vi "4_VisualAD_HyperParam_Search.vi"() -> ()   [LabVIEW 2020]
uses:
  <vilib>/Ngene/DeepLTK Anomaly Detection Addon/Toolkit/API/Controls/NNPC_Coreset_Params.ctl
  <vilib>/Ngene/DeepLTK Anomaly Detection Addon/Toolkit/API/Controls/Distance_Metric.ctl
  <vilib>/Ngene/DeepLTK Anomaly Detection Addon/Toolkit/API/Controls/NNPC_Setup.ctl
  <vilib>/Ngene/Deep Learning Toolkit/Toolkit/NN_Data/API/NN_Dims(C,H,W).ctl
  <vilib>/Ngene/Deep Learning Toolkit/Toolkit/NN_Network/Controls/NN_Device.ctl
  <vilib>/Ngene/DeepLTK Anomaly Detection Addon/Toolkit/API/Controls/Feature_Scorer_Params.ctl
  <vilib>/Ngene/DeepLTK Anomaly Detection Addon/Toolkit/API/Controls/Gaussian_Blur.ctl
  <vilib>/Ngene/DeepLTK Anomaly Detection Addon/Toolkit/API/Controls/Evaluation_Metrics.ctl
  <vilib>/Ngene/DeepLTK Anomaly Detection Addon/Toolkit/API/Controls/Eval_Results.ctl
  <vilib>/Ngene/DeepLTK Anomaly Detection Addon/Toolkit/API/Controls/MinMax.ctl
  <vilib>/Ngene/DeepLTK Anomaly Detection Addon/Toolkit/API/Controls/NNPC_Random_Projection_CFG.ctl
  <vilib>/Ngene/DeepLTK Anomaly Detection Addon/Toolkit/API/Controls/Dim_Reduction_Method.ctl
  <vilib>/Ngene/DeepLTK Anomaly Detection Addon/Toolkit/API/Controls/NNFE_CFG.ctl
  <vilib>/Ngene/DeepLTK Anomaly Detection Addon/Toolkit/API/Controls/Layer_Selector.ctl
  <vilib>/Ngene/DeepLTK Anomaly Detection Addon/Toolkit/API/Controls/Feature_Layer_Selector.ctl
  <vilib>/Ngene/DeepLTK Anomaly Detection Addon/Toolkit/API/Controls/Interpolation_Selector.ctl
  subVIs/HyperParam_Search/Controls/Feature_Layers_CFG.ctl
  subVIs/HyperParam_Search/Controls/Model_Info_and_Report.ctl
  subVIs/Dataset_Reader/Controls/Read_Options.ctl
  <vilib>/Ngene/DeepLTK Anomaly Detection Addon/Toolkit/API/Controls/NNPC_PreProcessing_Options.ctl
  <vilib>/Ngene/DeepLTK Anomaly Detection Addon/Toolkit/API/Controls/Crop_CFG.ctl
  <vilib>/Ngene/DeepLTK Anomaly Detection Addon/Toolkit/API/Controls/NNPC_DS_Stats.ctl
  <vilib>/Ngene/DeepLTK Anomaly Detection Addon/Toolkit/API/Controls/Image_Stats_RGB.ctl
  <vilib>/Ngene/DeepLTK Anomaly Detection Addon/Toolkit/API/Controls/Eval_Config.ctl
  <vilib>/Ngene/DeepLTK Anomaly Detection Addon/Toolkit/API/NNPC_Generate_Embedding/NNPC_Generate_Embedding(Dataset).vi
  <vilib>/Ngene/DeepLTK Anomaly Detection Addon/Toolkit/API/NNPC_Predict/NNPC_Predict(Dataset).vi
  <vilib>/Ngene/Deep Learning Toolkit/Toolkit/NN_Data/subVIs/Dataset_Destroy/NN_Dataset_Destroy(In3D_Out3D).vi
  <vilib>/Ngene/DeepLTK Anomaly Detection Addon/Toolkit/DeepLTK_Anomaly_Detection_Addon.lvlib
  <vilib>/Ngene/Deep Learning Toolkit/Toolkit/Deep_Learning_Toolkit_by_Ngene.lvlib
panel:
  in  "Model_Info_and_Report":T1={"Idx"=0, "Name"="", "Feature Extractor"="wrn_50_2_2_bnmerge", "Layers"="", "DS_Size"=0, "H"=0, "W"=-1, "Coreset Size"=0, "Proj_Dim"=0, "Good_Max(Img)"=0.0, "Bad_Min(Img)"=0.0, "Rel_Margin"=0.0, "Image_AUC"=0.0, "Pixel_AUC"=0.0, "Image_F1_Max"=0.0, "Pixel_F1_Max"=0.0, "Train_Time"=0.0, "Inf_Time"=0.0} {"Rel_Margin" format="%#.5f"; "Bad_Min(Img)" format="%#.5f"; "Good_Max(Img)" format="%#.5f"; "Pixel_F1_Max" format="%#.5f"; "Pixel_AUC" format="%#.5f"; "Image_F1_Max" format="%#.5f"; "Image_AUC" format="%#.5f"}
  in  "Tab Control":enum32{"Setup", "Results"}(tab)
  in  "Min_Layers_In_Group":u16=1
  in  "Dataset_Path(Train/Test/GT)":path=path "D:/Ngene/GitHub/deepltk_examples/3_Image_Processing/36_Anomaly_Detection/Dataset/Playing_Cards_3ofHearts"
  in  "Destination_Path":path=path "D:/working"
  in  "Coreset_Size":sgl[](array[numeric])=[5000.0, 10000.0, 15000.0]
  in  "Proj._Dim.":i32[](array[numeric])=[-1]
  in  "Coreset_Params":T2={"Distance_Metric"=enum."Euclidean", "CoreSet_Size"=1.0, "Start_idx"=3}
  in  "NNPC_Setup":T4={"Input_Dims"={"C"=3, "H"=224, "W"=224}, "mBatch"=1, "Device"=enum."GPU", "GPU Id"=0}
  in  "Feature_Scorer_Params":T7={"Nearest_Neighbors"=1, "Calculate Anomaly Map"=FALSE, "Gaussian_Blur"={"Kernel_Size"=33, "Sigma"=4.0}}
  in  "Dim Reduction":T9={"Method"=enum."Rnd_Proj", "Target_Dim"=-1, "Seed"=42}
  in  "NNFE_CFG":T11={"Name"="Cards_3ofHearts", "Layer_Selection_By"=enum."Stride", "Feature_Layers"={"[LayerID, PatchSize]"=[{"Layer_ID"=8, "Patch_Size"=3}, {"Layer_ID"=16, "Patch_Size"=3}]}, "Interpolation_Type"=enum."Bi-Linear"}
  in  "NNFE_Folder_Paths":path[](array[path])=[path "D:/Ngene/GitHub/deepltk_examples/3_Image_Processing/36_Anomaly_Detection/NNFE/WRN_50_2_2_L3"]
  in  "Patch Sizes":i32[](array[numeric])=[1, 3, 5]
  in  "Layer ID":i32[](array[numeric])=[4, 8, 16]
  out "Generated_Feature_Layers":T13[](array[typedef])=[{"[LayerID, PatchSize]"=[{"Layer_ID"=16, "Patch_Size"=1}]}, {"[LayerID, PatchSize]"=[{"Layer_ID"=16, "Patch_Size"=3}]}, {"[LayerID, PatchSize]"=[{"Layer_ID"=16, "Patch_Size"=5}]}, {"[LayerID, PatchSize]"=[{"Layer_ID"=8, "Patch_Size"=1}]}, {"[LayerID, PatchSize]"=[{"Layer_ID"=8, "Patch_Size"=1}, {"Layer_ID"=16, "Patch_Size"=1}]}, {"[LayerID, PatchSize]"=[{"Layer_ID"=8, "Patch_Size"=1}, {"Layer_ID"=16, "Patch_Size"=3}]}, {"[LayerID, PatchSize]"=[{"Layer_ID"=8, "Patch_Size"=1}, {"Layer_ID"=16, "Patch_Size"=5}]}, {"[LayerID, PatchSize]"=[{"Layer_ID"=8, "Patch_Size"=3}]}, {"[LayerID, PatchSize]"=[{"Layer_ID"=8, "Patch_Size"=3}, {"Layer_ID"=16, "Patch_Size"=1}]}, {"[LayerID, PatchSize]"=[{"Layer_ID"=8, "Patch_Size"=3}, {"Layer_ID"=16, "Patch_Size"=3}]}, {"[LayerID, PatchSize]"=[{"Layer_ID"=8, "Patch_Size"=3}, {"Layer_ID"=16, "Patch_Size"=5}]}, {"[LayerID, PatchSize]"=[{"Layer_ID"=8, "Patch_Size"=5}]}, {"[LayerID, PatchSize]"=[{"Layer_ID"=8, "Patch_Size"=5}, {"Layer_ID"=16, "Patch_Size"=1}]}, {"[LayerID, PatchSize]"=[{"Layer_ID"=8, "Patch_Size"=5}, {"Layer_ID"=16, "Patch_Size"=3}]}, {"[LayerID, PatchSize]"=[{"Layer_ID"=8, "Patch_Size"=5}, {"Layer_ID"=16, "Patch_Size"=5}]}, {"[LayerID, PatchSize]"=[{"Layer_ID"=4, "Patch_Size"=1}]}, {"[LayerID, PatchSize]"=[{"Layer_ID"=4, "Patch_Size"=1}, {"Layer_ID"=16, "Patch_Size"=1}]}, {"[LayerID, PatchSize]"=[{"Layer_ID"=4, "Patch_Size"=1}, {"Layer_ID"=16, "Patch_Size"=3}]}, {"[LayerID, PatchSize]"=[{"Layer_ID"=4, "Patch_Size"=1}, {"Layer_ID"=16, "Patch_Size"=5}]}, {"[LayerID, PatchSize]"=[{"Layer_ID"=4, "Patch_Size"=1}, {"Layer_ID"=8, "Patch_Size"=1}]}, {"[LayerID, PatchSize]"=[{"Layer_ID"=4, "Patch_Size"=1}, {"Layer_ID"=8, "Patch_Size"=3}]}, {"[LayerID, PatchSize]"=[{"Layer_ID"=4, "Patch_Size"=1}, {"Layer_ID"=8, "Patch_Size"=5}]}, {"[LayerID, PatchSize]"=[{"Layer_ID"=4, "Patch_Size"=3}]}, {"[LayerID, PatchSize]"=[{"Layer_ID"=4, "Patch_Size"=3}, {"Layer_ID"=16, "Patch_Size"=1}]}, {"[LayerID, PatchSize]"=[{"Layer_ID"=4, "Patch_Size"=3}, {"Layer_ID"=16, "Patch_Size"=3}]}, {"[LayerID, PatchSize]"=[{"Layer_ID"=4, "Patch_Size"=3}, {"Layer_ID"=16, "Patch_Size"=5}]}, {"[LayerID, PatchSize]"=[{"Layer_ID"=4, "Patch_Size"=3}, {"Layer_ID"=8, "Patch_Size"=1}]}, {"[LayerID, PatchSize]"=[{"Layer_ID"=4, "Patch_Size"=3}, {"Layer_ID"=8, "Patch_Size"=3}]}, {"[LayerID, PatchSize]"=[{"Layer_ID"=4, "Patch_Size"=3}, {"Layer_ID"=8, "Patch_Size"=5}]}, {"[LayerID, PatchSize]"=[{"Layer_ID"=4, "Patch_Size"=5}]}, {"[LayerID, PatchSize]"=[{"Layer_ID"=4, "Patch_Size"=5}, {"Layer_ID"=16, "Patch_Size"=1}]}, {"[LayerID, PatchSize]"=[{"Layer_ID"=4, "Patch_Size"=5}, {"Layer_ID"=16, "Patch_Size"=3}]}, {"[LayerID, PatchSize]"=[{"Layer_ID"=4, "Patch_Size"=5}, {"Layer_ID"=16, "Patch_Size"=5}]}, {"[LayerID, PatchSize]"=[{"Layer_ID"=4, "Patch_Size"=5}, {"Layer_ID"=8, "Patch_Size"=1}]}, {"[LayerID, PatchSize]"=[{"Layer_ID"=4, "Patch_Size"=5}, {"Layer_ID"=8, "Patch_Size"=3}]}, {"[LayerID, PatchSize]"=[{"Layer_ID"=4, "Patch_Size"=5}, {"Layer_ID"=8, "Patch_Size"=5}]}]
  in  "Max_Layers_In_Group":u16=2
  out "error out":errorcluster
  in  "Img Res. H":i32[](array[numeric])=[224, 368]
  in  "Img Res. W":i32[](array[numeric])=[224, 368]
  in  "Single DS?":bool=TRUE
  out "Img._W":i32=224
  out "Elapsed Time":dbl=22.38694479999998 format="%<%H:%M:%S>t"
  out "Max_Dist":sgl[](graph)
  out "Tot Itr of one DS":i32=216
  out "Current Iter":i32=12
  out "Coreset Size":i32=3
  out "Proj. Dim.":i32=1
  out "Img Res.":i32=2
  out "Feature_Layers":i32=36
  out "Elapsed Time":dbl=22.38694479999998
  out "Evaluation_Metrics(Image)":T15={"Scores(Good)"={"X Values"=[56.569074115753175, 56.90936315536499, 57.249652194976804, 57.58994123458862, 57.93023027420044, 58.27051931381226, 58.610808353424076, 58.95109739303589, 59.291386432647705, 59.63167547225952, 59.971964511871334, 60.31225355148315, 60.65254259109497, 60.99283163070679, 61.33312067031861, 61.67340970993042, 62.013698749542236, 62.353987789154054, 62.694276828765865, 63.03456586837768, 63.3748549079895, 63.71514394760132, 64.05543298721314, 64.39572202682496, 64.73601106643676, 65.07630010604859, 65.4165891456604, 65.75687818527223, 66.09716722488403, 66.43745626449585, 66.77774530410767, 67.11803434371947, 67.4583233833313, 67.79861242294311, 68.13890146255494, 68.47919050216674, 68.81947954177856, 69.15976858139038, 69.50005762100218, 69.84034666061402, 70.18063570022582, 70.52092473983765, 70.86121377944946, 71.20150281906129, 71.5417918586731, 71.88208089828491, 72.22236993789673, 72.56265897750853, 72.90294801712037, 73.24323705673217, 73.583526096344, 73.9238151359558, 74.26410417556762, 74.60439321517944, 74.94468225479126, 75.28497129440308, 75.62526033401488, 75.96554937362671, 76.30583841323852, 76.64612745285035, 76.98641649246215, 77.32670553207397, 77.66699457168579, 78.0072836112976, 78.34757265090943, 78.68786169052123, 79.02815073013306, 79.36843976974487, 79.7087288093567, 80.0490178489685, 80.38930688858032, 80.72959592819214, 81.06988496780394, 81.41017400741578, 81.75046304702758, 82.09075208663941, 82.43104112625122, 82.77133016586303, 83.11161920547485, 83.45190824508667, 83.79219728469849, 84.13248632431029, 84.47277536392212, 84.81306440353393, 85.15335344314576, 85.49364248275756, 85.83393152236938, 86.1742205619812, 86.514509601593, 86.85479864120484, 87.19508768081664, 87.53537672042847, 87.87566576004028, 88.2159547996521, 88.55624383926391, 88.89653287887573, 89.23682191848755, 89.57711095809937, 89.91739999771119, 90.25768903732299], "Histogram: h(x)"=[3, 0, 0, 0, 1, 0, 1, 1, 1, 2, 1, 0, 0, 1, 0, 0, 3, 2, 0, 0, 0, 1, 0, 1, 0, 0, 0, 0, 0, 0, 0, 0, 0, 0, 0, 0, 0, 0, 0, 0, 0, 0, 0, 1, 1, 0, 0, 0, 0, 0, 0, 0, 0, 0, 0, 0, 0, 0, 0, 1, 0, 0, 0, 0, 0, 0, 0, 0, 0, 1, 0, 0, 0, 0, 0, 0, 0, 0, 0, 0, 0, 1, 1, 0, 0, 1, 0, 0, 0, 0, 0, 0, 0, 0, 0, 0, 0, 0, 0, 0]}, "Scores(Bad)"={"X Values"=[56.569074115753175, 56.90936315536499, 57.249652194976804, 57.58994123458862, 57.93023027420044, 58.27051931381226, 58.610808353424076, 58.95109739303589, 59.291386432647705, 59.63167547225952, 59.971964511871334, 60.31225355148315, 60.65254259109497, 60.99283163070679, 61.33312067031861, 61.67340970993042, 62.013698749542236, 62.353987789154054, 62.694276828765865, 63.03456586837768, 63.3748549079895, 63.71514394760132, 64.05543298721314, 64.39572202682496, 64.73601106643676, 65.07630010604859, 65.4165891456604, 65.75687818527223, 66.09716722488403, 66.43745626449585, 66.77774530410767, 67.11803434371947, 67.4583233833313, 67.79861242294311, 68.13890146255494, 68.47919050216674, 68.81947954177856, 69.15976858139038, 69.50005762100218, 69.84034666061402, 70.18063570022582, 70.52092473983765, 70.86121377944946, 71.20150281906129, 71.5417918586731, 71.88208089828491, 72.22236993789673, 72.56265897750853, 72.90294801712037, 73.24323705673217, 73.583526096344, 73.9238151359558, 74.26410417556762, 74.60439321517944, 74.94468225479126, 75.28497129440308, 75.62526033401488, 75.96554937362671, 76.30583841323852, 76.64612745285035, 76.98641649246215, 77.32670553207397, 77.66699457168579, 78.0072836112976, 78.34757265090943, 78.68786169052123, 79.02815073013306, 79.36843976974487, 79.7087288093567, 80.0490178489685, 80.38930688858032, 80.72959592819214, 81.06988496780394, 81.41017400741578, 81.75046304702758, 82.09075208663941, 82.43104112625122, 82.77133016586303, 83.11161920547485, 83.45190824508667, 83.79219728469849, 84.13248632431029, 84.47277536392212, 84.81306440353393, 85.15335344314576, 85.49364248275756, 85.83393152236938, 86.1742205619812, 86.514509601593, 86.85479864120484, 87.19508768081664, 87.53537672042847, 87.87566576004028, 88.2159547996521, 88.55624383926391, 88.89653287887573, 89.23682191848755, 89.57711095809937, 89.91739999771119, 90.25768903732299], "Histogram: h(x)"=[0, 0, 0, 0, 0, 0, 0, 0, 0, 0, 0, 0, 0, 0, 0, 0, 0, 0, 0, 0, 0, 0, 0, 0, 0, 0, 0, 0, 0, 0, 0, 0, 0, 0, 0, 0, 0, 0, 0, 0, 0, 0, 0, 0, 0, 0, 0, 0, 0, 0, 0, 0, 0, 0, 0, 0, 0, 0, 0, 0, 0, 0, 1, 0, 0, 0, 1, 0, 0, 2, 0, 0, 3, 1, 2, 0, 2, 0, 1, 1, 1, 0, 2, 3, 2, 1, 0, 0, 0, 1, 0, 0, 0, 0, 0, 0, 0, 0, 0, 1]}, "Eval Stats"={"Scores(Good)"={"Min"=56.39893, "Max"=85.355675}, "Scores(Bad)"={"Min"=77.81394, "Max"=90.42783}, "# of Samples(Good)"=25, "# of Samples(Bad)"=25, "AUROC"=0.9096, "F1_Max"=0.92592597, "Thrshld(F1_Max)"=76.63233, "Prec.(F1_Max)"=0.86206895, "Recall(F1_Max)"=1.0, "FPR(F1_Max)"=0.16, "FNR(F1_Max)"=0.0}} {"Eval Stats"."Recall(F1_Max)" format="%#.5f"; "Eval Stats"."FPR(F1_Max)" format="%#.5f"; "Eval Stats"."FNR(F1_Max)" format="%#.5f"; "Eval Stats"."Prec.(F1_Max)" format="%#.5f"; "Eval Stats"."F1_Max" format="%#.5f"; "Eval Stats"."AUROC" format="%#.5f"; "Eval Stats"."Scores(Bad)"."Min" format="%#_5g"; "Eval Stats"."Scores(Good)"."Min" format="%#_5g"; "Eval Stats"."Thrshld(F1_Max)" format="%#_5f"}
  out "Evaluation_Metrics(Pixel)":T15={"Scores(Good)"={"X Values"=[0.0, 0.0, 0.0, 0.0, 0.0, 0.0, 0.0, 0.0, 0.0, 0.0, 0.0, 0.0, 0.0, 0.0, 0.0, 0.0, 0.0, 0.0, 0.0, 0.0, 0.0, 0.0, 0.0, 0.0, 0.0, 0.0, 0.0, 0.0, 0.0, 0.0, 0.0, 0.0, 0.0, 0.0, 0.0, 0.0, 0.0, 0.0, 0.0, 0.0, 0.0, 0.0, 0.0, 0.0, 0.0, 0.0, 0.0, 0.0, 0.0, 0.0, 0.0, 0.0, 0.0, 0.0, 0.0, 0.0, 0.0, 0.0, 0.0, 0.0, 0.0, 0.0, 0.0, 0.0, 0.0, 0.0, 0.0, 0.0, 0.0, 0.0, 0.0, 0.0, 0.0, 0.0, 0.0, 0.0, 0.0, 0.0, 0.0, 0.0, 0.0, 0.0, 0.0, 0.0, 0.0, 0.0, 0.0, 0.0, 0.0, 0.0, 0.0, 0.0, 0.0, 0.0, 0.0, 0.0, 0.0, 0.0, 0.0, 0.0], "Histogram: h(x)"=[]}, "Scores(Bad)"={"X Values"=[], "Histogram: h(x)"=[]}, "Eval Stats"={"Scores(Good)"={"Min"=0.0, "Max"=0.0}, "Scores(Bad)"={"Min"=0.0, "Max"=0.0}, "# of Samples(Good)"=0, "# of Samples(Bad)"=0, "AUROC"=-1.0, "F1_Max"=0.0, "Thrshld(F1_Max)"=0.0, "Prec.(F1_Max)"=0.0, "Recall(F1_Max)"=0.0, "FPR(F1_Max)"=0.0, "FNR(F1_Max)"=0.0}} {"Eval Stats"."Recall(F1_Max)" format="%#.5f"; "Eval Stats"."FPR(F1_Max)" format="%#.5f"; "Eval Stats"."FNR(F1_Max)" format="%#.5f"; "Eval Stats"."Prec.(F1_Max)" format="%#.5f"; "Eval Stats"."F1_Max" format="%#.5f"; "Eval Stats"."AUROC" format="%#.5f"; "Eval Stats"."Scores(Bad)"."Min" format="%#_5g"; "Eval Stats"."Scores(Good)"."Min" format="%#_5g"; "Eval Stats"."Thrshld(F1_Max)" format="%#_5f"}
  out "Coreset Size":i32
  out "Coreset Size":i32=15000
  out "Proj. Dim.":i32=-1
  out "Img._H":i32=224
  out "Proj. Dim.":i32
  out "Img Res.":i32
  out "dT_Eval":dbl=0.00020089999998162966 format="%#_4p"
  out "dT_Inference":dbl=0.007889208000001417 format="%#_4p"
  out "dT_Coreset":dbl=11.027360000000044 format="%#_4p"
  out "dT_Embed":dbl=0.20192650000001322 format="%#_3p"
  out "dT_Init":dbl=0.13968869999996514 format="%#_3p"
  out "dT_DS_Read(Test)":dbl=0.14549890000000687 format="%#_3p"
  out "dT_DS_Read(Train)":dbl=0.19376790000001165 format="%#_3p"
  out "DS Size(Test)":i32=50
  out "DS Size(Train)":i32=50
  out "Feature_Layers":i32=4
  out "dT_DS_Read(Train)":dbl=0.19376790000001165 format="%#.0f"
  out "dT_DS_Read(Test)":dbl=0.14549890000000687 format="%#.0f"
  out "dT_Init":dbl=1.64397120000001 format="%#.0f"
  out "dT_Predict":dbl=2.67796850000002 format="%#.0f"
  out "dT_Coreset":dbl=16.00583629999994 format="%#.0f"
  out "dT_Embed":dbl=0.9169715000000451 format="%#.0f"
  out "dT_Eval":dbl=0.0023649000001455533 format="%#.0f"
  out "Feature Extractor":string="wrn_50_2_2_bnmerge"
  out "dT_Predict":dbl=0.3944604000000709 format="%#_5p"
  out "[LayerID, PatchSize]":T18=[{"Layer_ID"=8, "Patch_Size"=1}, {"Layer_ID"=16, "Patch_Size"=1}]
  in  "Stop":bool
  out "NNFE":i32
  out "NNFE":i32=1
  out "Best_Model":string="9_wrn_50_2_2_bnmerge_Res224x224_L8P1_Prj-1_CSet15k"
  out "Best_AUC":sgl=0.9696 format="%#_5g"
  out "DS":i32=1
  out "DS":i32
  out "DS_Name":string="Playing_Cards_3ofHearts"
  out "Crrnt Iter":i32=12
  out "Total Iters":i32=216
  out "Online_CoreSet_Size":sgl=-1.0 format="%#_4g"
  # "Total Iterations"
  # "Current Iteration"
  # "Current Settings"
  # "Total Times"
  # "Best Settings"
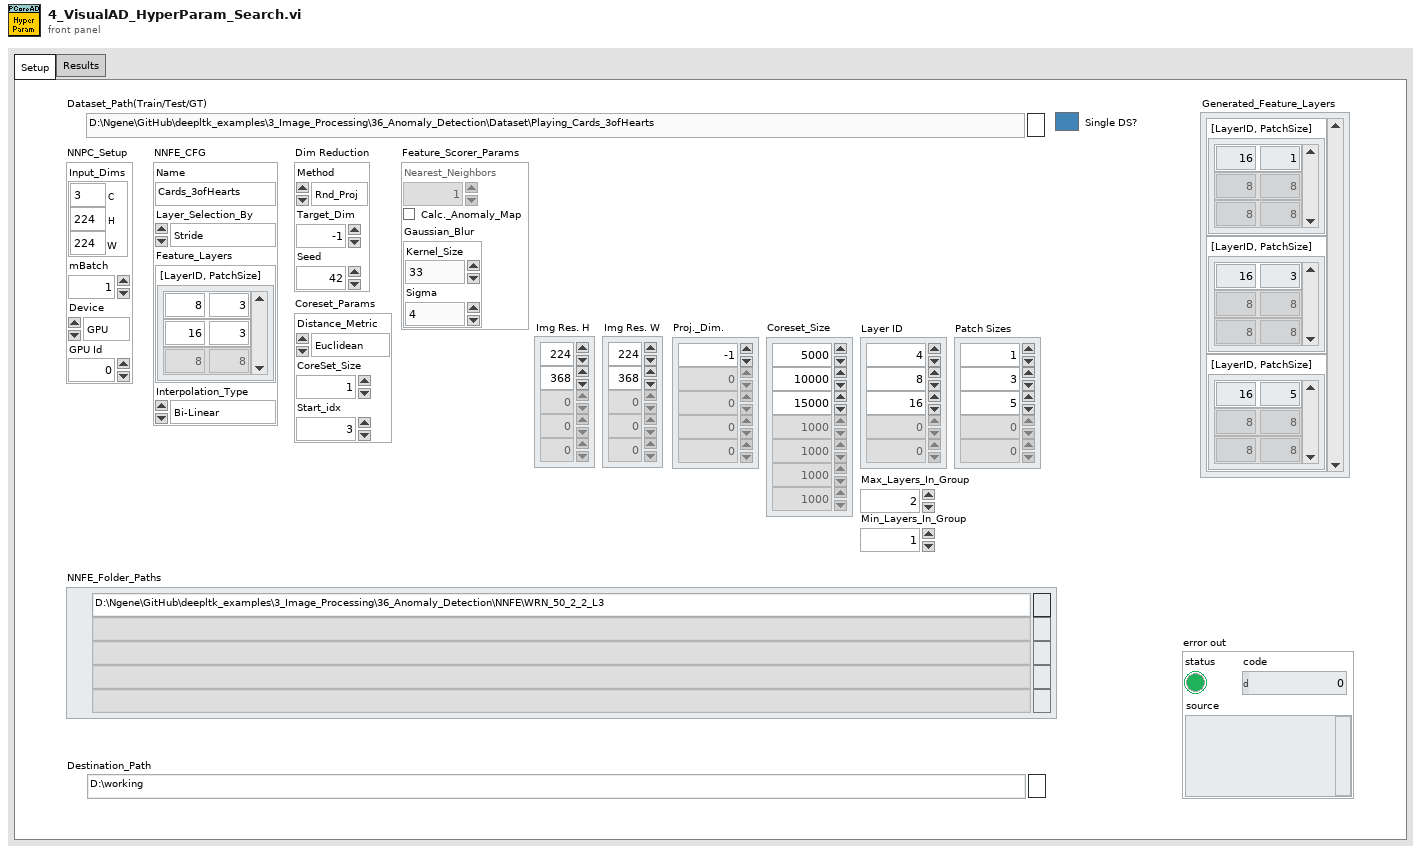
[diagram p1: front panel]
types:
  T1 = typedef "Model_Info_and_Report.ctl" = cluster{"Idx":i32, "Name":string, "Feature Extractor":string, "Layers":string, "DS_Size":i32, "H":i32, "W":i32, "Coreset Size":i32, "Proj_Dim":i32, "Good_Max(Img)":sgl, "Bad_Min(Img)":sgl, "Rel_Margin":sgl, "Image_AUC":sgl, "Pixel_AUC":sgl, "Image_F1_Max":sgl, "Pixel_F1_Max":sgl, "Train_Time":dbl, "Inf_Time":dbl}
  T2 = typedef "DeepLTK_Anomaly_Detection_Addon.lvlib/NNPC_Coreset_Params.ctl" = cluster{"Distance_Metric":T3, "CoreSet_Size":sgl, "Start_idx":i32}
  T3 = typedef "DeepLTK_Anomaly_Detection_Addon.lvlib/Distance_Metric.ctl" = enum16{"Euclidean", "Cosine"}
  T4 = typedef "DeepLTK_Anomaly_Detection_Addon.lvlib/NNPC_Setup.ctl" = cluster{"Input_Dims":T5, "mBatch":i32, "Device":T6, "GPU Id":i32}
  T5 = typedef "Deep_Learning_Toolkit_by_Ngene.lvlib/NN_Dims(C,H,W).ctl" = cluster{"C":i32, "H":i32, "W":i32}
  T6 = typedef "Deep_Learning_Toolkit_by_Ngene.lvlib/NN_Device.ctl" = enum16{"CPU", "GPU"}
  T7 = typedef "DeepLTK_Anomaly_Detection_Addon.lvlib/Feature_Scorer_Params.ctl" = cluster{"Nearest_Neighbors":i32, "Calculate Anomaly Map":bool, "Gaussian_Blur":T8}
  T8 = typedef "DeepLTK_Anomaly_Detection_Addon.lvlib/Gaussian_Blur.ctl" = cluster{"Kernel_Size":i32, "Sigma":sgl}
  T9 = typedef "DeepLTK_Anomaly_Detection_Addon.lvlib/NNPC_Random_Projection_CFG.ctl" = cluster{"Method":T10, "Target_Dim":i32, "Seed":i32}
  T10 = typedef "DeepLTK_Anomaly_Detection_Addon.lvlib/Dim_Reduction_Method.ctl" = enum16{"None", "Rnd_Proj", "PCA"}
  T11 = typedef "DeepLTK_Anomaly_Detection_Addon.lvlib/NNFE_CFG.ctl" = cluster{"Name":string, "Layer_Selection_By":T12, "Feature_Layers":T13, "Interpolation_Type":T14}
  T12 = typedef "DeepLTK_Anomaly_Detection_Addon.lvlib/Layer_Selector.ctl" = enum16{"Stride", "Layer_Idx"}
  T13 = typedef "DeepLTK_Anomaly_Detection_Addon.lvlib/Feature_Layer_Selector.ctl" = cluster{"[LayerID, PatchSize]":cluster{"Layer_ID":i32, "Patch_Size":i32}[]}
  T14 = typedef "DeepLTK_Anomaly_Detection_Addon.lvlib/Interpolation_Selector.ctl" = enum16{"Nearest", "Bi-Linear"}
  T15 = typedef "DeepLTK_Anomaly_Detection_Addon.lvlib/Evaluation_Metrics.ctl" = cluster{"Scores(Good)":cluster{"X Values":dbl[], "Histogram: h(x)":i32[]}, "Scores(Bad)":cluster{"X Values":dbl[], "Histogram: h(x)":i32[]}, "Eval Stats":T16}
  T16 = typedef "DeepLTK_Anomaly_Detection_Addon.lvlib/Eval_Results.ctl" = cluster{"Scores(Good)":T17, "Scores(Bad)":T17, "# of Samples(Good)":i32, "# of Samples(Bad)":i32, "AUROC":sgl, "F1_Max":sgl, "Thrshld(F1_Max)":sgl, "Prec.(F1_Max)":sgl, "Recall(F1_Max)":sgl, "FPR(F1_Max)":sgl, "FNR(F1_Max)":sgl}
  T17 = typedef "DeepLTK_Anomaly_Detection_Addon.lvlib/MinMax.ctl" = cluster{"Min":sgl, "Max":sgl}
  T18 = typedef "Feature_Layers_CFG.ctl" = cluster{"Layer_ID":i32, "Patch_Size":i32}[]
  T19 = typedef "DeepLTK_Anomaly_Detection_Addon.lvlib/NN_Paths.ctl" = cluster{"CFG":path, "BIN":path}
  T20 = enum16{"open", "replace", "create", "open or create", "replace or create", "replace or create with confirmation"}
  T21 = typedef "DeepLTK_Anomaly_Detection_Addon.lvlib/NNPC_PreProcessing_Options.ctl" = cluster{"DS_Name":string, "Input_Dims":T5, "Cropping":T22, "Interpolation Type":u32, "MultiStage_ReSample?":bool, "Dataset_Stats":T23}
  T22 = typedef "DeepLTK_Anomaly_Detection_Addon.lvlib/Crop_CFG.ctl" = cluster{"Left":sgl, "Top":sgl, "Right":sgl, "Bottom":sgl}
  T23 = typedef "DeepLTK_Anomaly_Detection_Addon.lvlib/NNPC_DS_Stats.ctl" = cluster{"means":T24, "stds":T24}
  T24 = typedef "DeepLTK_Anomaly_Detection_Addon.lvlib/Image_Stats_RGB.ctl" = cluster{"R":sgl, "G":sgl, "B":sgl}
  T25 = typedef "Read_Options.ctl" = cluster{"Read Bads?":bool, "Read GTs?":bool, "Update. DS Stats?":bool}
  T26 = typedef "DeepLTK_Anomaly_Detection_Addon.lvlib/Eval_Config.ctl" = cluster{"Extract_Good_Pixels_from_Bad":bool, "# bins":i32}
  T27 = typedef "Deep_Learning_Toolkit_by_Ngene.lvlib/NN_DataSet(In3D_Out3D).ctl" = cluster{"Dataset_Size":i32, "Dims_In":T5, "Labels":string[], "File Paths":path[], "Outputs Ref.":T28, "Inputs Ref.":variant, "Dims_Out":T5, "Custom_Data":variant}
  T28 = typedef "Deep_Learning_Toolkit_by_Ngene.lvlib/NN_Data_ref(4D_SGL).ctl" = refnum<data-value>
  T29 = typedef "DeepLTK_Anomaly_Detection_Addon.lvlib/NNPC_Instance.ctl" = cluster{"Name":string, "NN":T30, "MemBank_Data":T44}
  T30 = typedef "Deep_Learning_Toolkit_by_Ngene.lvlib/NN.ctl" = cluster{"Name":string, "No of Layers":i32, "mBatch":i32, "Layers":T31[], "Dimty":T32, "Dims_In":T5, "Dims_Out":T5, "Working_Dir":path, "Train?":bool, "Train_Params":T33, "LR_Update_Policy":T36, "Session Data":T38, "Ground_truth":T39, "NNg_hdls":T40, "NN_Device":T6, "GPU Id":i32, "Labels":string[], "Loss_Type":T41, "Loss_Cfg_Prms":variant, "NNG_WS":T42, "DryRun?":bool}
  T31 = typedef "Deep_Learning_Toolkit_by_Ngene.lvlib/NN_Layer_ref.ctl" = refnum<file>
  T32 = typedef "Deep_Learning_Toolkit_by_Ngene.lvlib/NN_In_Out_Dim-ty.ctl" = enum8{"In1D_Out1D", "In3D_Out1D", "In3D_Out3D", "In3D_OutBBox"}
  T33 = typedef "Deep_Learning_Toolkit_by_Ngene.lvlib/NN_Train_Params.ctl" = cluster{"Optimizer":T34, "Beta_1":sgl, "Beta_2":sgl, "Weight Decay(L1)":sgl, "Weight Decay(L2)":sgl, "Data_Sampling":T35}
  T34 = typedef "Deep_Learning_Toolkit_by_Ngene.lvlib/NN_Train_Optimizer.ctl" = enum16{"SGD", "Adam", "Adagrad", "Adadelta", "RMSProp", "Nesterov"}
  T35 = typedef "Deep_Learning_Toolkit_by_Ngene.lvlib/NN_Train_Data_Sampling.ctl" = enum16{"Random", "Sequential"}
  T36 = typedef "Deep_Learning_Toolkit_by_Ngene.lvlib/NN_LR_Policy_Cfg.ctl" = cluster{"Policy_Type":T37, "LR0":dbl, "k":sgl, "WarmUp_Policy":enum16{"Step", "Ramp"}, "WarmUp_Iter":i32, "WarmUp_Ratio":sgl}
  T37 = typedef "Deep_Learning_Toolkit_by_Ngene.lvlib/NN_LR_Policy_Type.ctl" = enum16{"Manual", "Step", "Exp", "1/t"}
  T38 = typedef "Deep_Learning_Toolkit_by_Ngene.lvlib/NN_Train_Session_Data.ctl" = cluster{"Epochs":sgl, "Tot_Iter":i32, "LR":sgl, "LR_iter":i32}
  T39 = typedef "Deep_Learning_Toolkit_by_Ngene.lvlib/NN_Ground_truth.ctl" = cluster{"Y":variant}
  T40 = typedef "Deep_Learning_Toolkit_by_Ngene.lvlib/nng_cuda_handles.ctl" = cluster{"cudnn":u64, "cublas":u64, "stream":u64, "curand":u64}
  T41 = typedef "Deep_Learning_Toolkit_by_Ngene.lvlib/NN_Loss_Type.ctl" = enum16{"None", "MSE", "CrossEntropy", "YOLO_v2", "YOLO_v4"}
  T42 = typedef "Deep_Learning_Toolkit_by_Ngene.lvlib/NNG_WS.ctl" = cluster{"NNG_WS_Mem":T43, "Max_WS_Size":i64}
  T43 = typedef "Deep_Learning_Toolkit_by_Ngene.lvlib/NNg_WS_Mem_DVR.ctl" = refnum<data-value>
  T44 = typedef "DeepLTK_Anomaly_Detection_Addon.lvlib/MemBank_and_Norm_Variants.ctl" = cluster{"MemBank":variant, "MemBank Norm":variant}
  T45 = typedef "DeepLTK_Anomaly_Detection_Addon.lvlib/Evaluation_Metrics(Pixel_Image).ctl" = cluster{"Evaluation_Metrics(Pixel)":T15, "Evaluation_Metrics(Image)":T15}
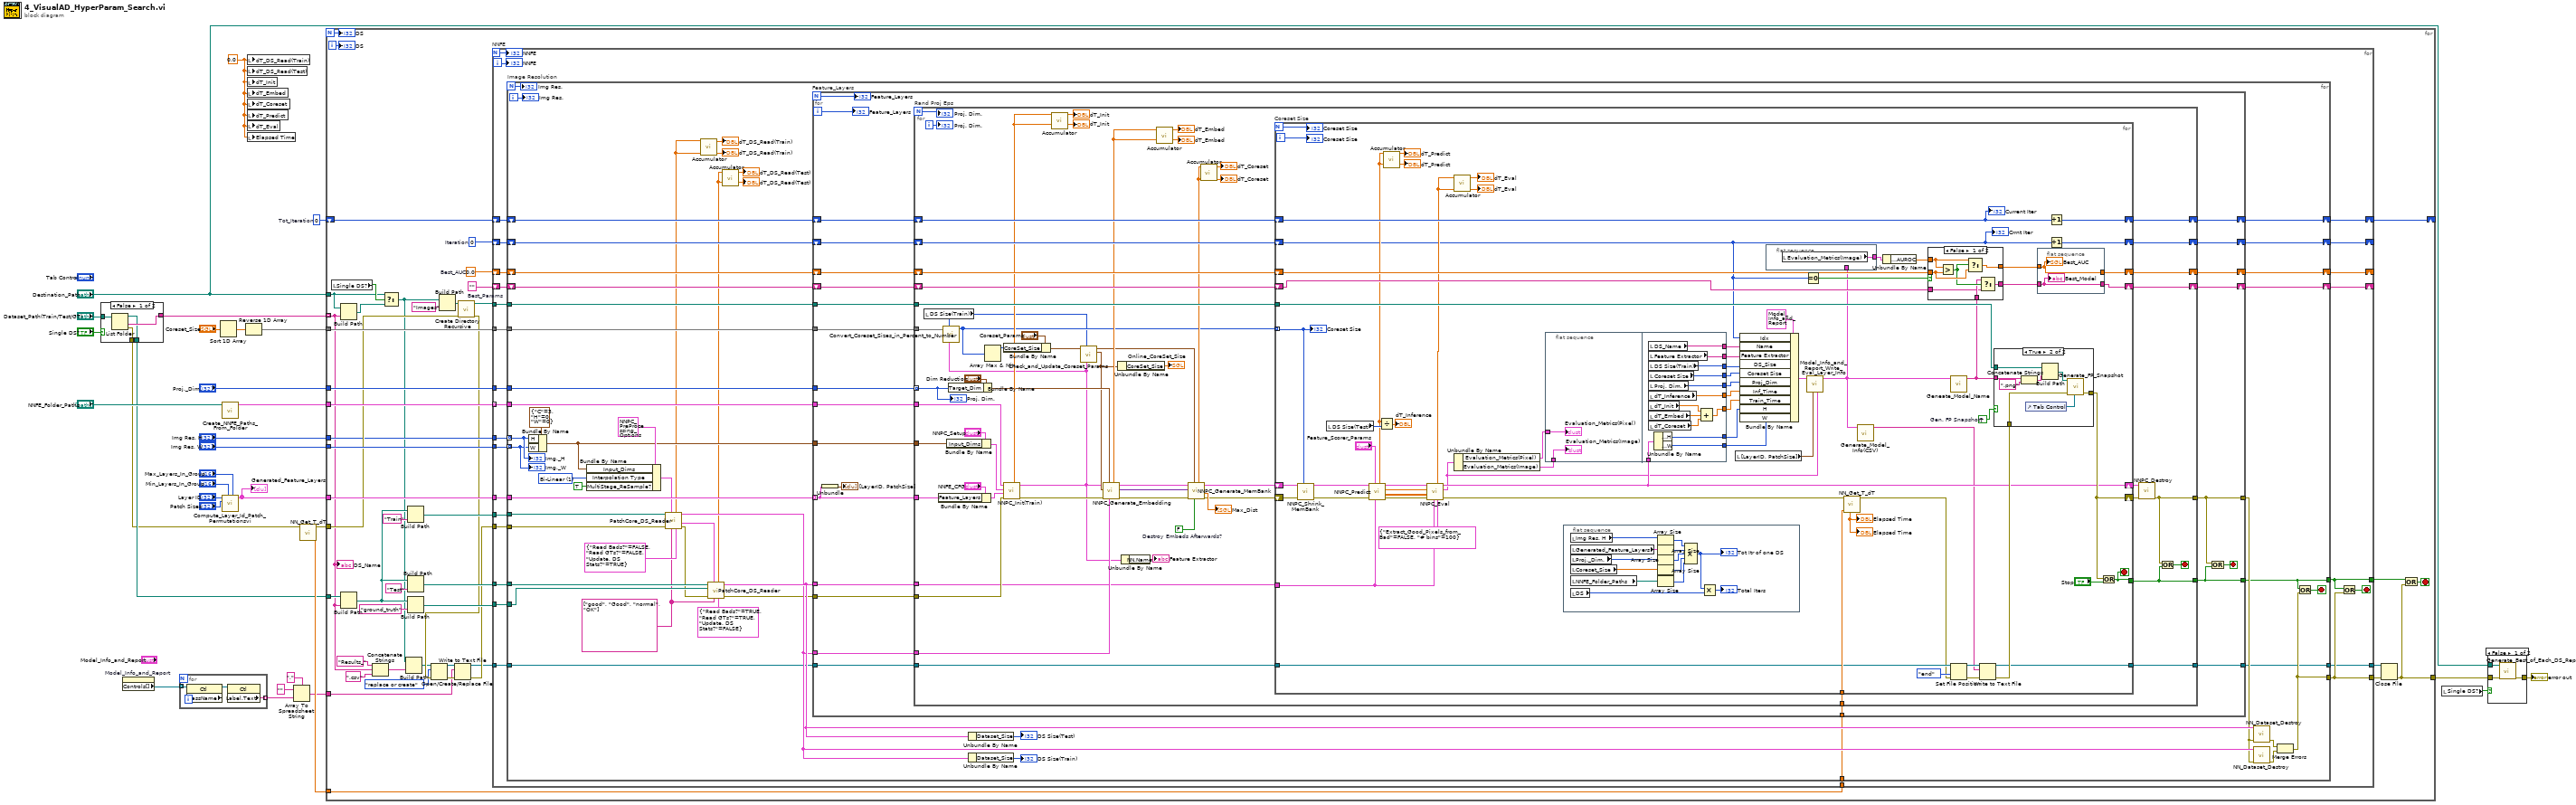
[diagram p0: block diagram]
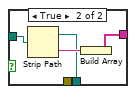
[diagram p4: hidden frame]
diagram:
  w10 = 0.0 ("dT_Eval")
  w20 = 0  # Tot_Iteration
  n1 = case shown="False" "Single DS?" {
    tunnel: "Dataset_Path(Train/Test/GT)" -> [w32 w37]
    tunnel: [w35 w38] -> w13
    tunnel: [w34 w36] -> w12
    tunnel: [w33 _] -> w11
    frame False {
      n2 = List Folder(path=w32) -> (path out=w34:path, folder names=w35:string[], error out=w33:errorcluster)  [unwired: 3 in, 1 out]
    }
    frame True {
      n3 = Strip Path(path=w37) -> (stripped path=w36:path, name=w39:string)
      n4 = Build Array(w39) -> (w38:string[])
    }
  }
  n5 = property on="Model_Info_and_Report" class="Clust (strict)"() -> ("Controls[]"=w6:refnum<vi>[])  [unwired: 2 in, 2 out]
  n6 = for {
    tunnel: w6 -> [w42] mode=indexing
    tunnel: [w40] -> w5 mode=indexing
    n7 = property class="Ctl" props=["ClassName"](reference=w42) -> (reference out=w41:refnum<vi>)  [unwired: 1 in, 2 out]
    n8 = property class="Ctl"(reference=w41) -> ("Label.Text"=w40:string)  [unwired: 1 in, 2 out]
  }
  n9 = Sort 1D Array(array="Coreset_Size") -> (sorted array=w29:sgl[])
  n10 = call "Create_NNFE_Paths_From_Folder.vi"("NNFE_Folder_Paths"="NNFE_Folder_Paths") -> ("NNFE_File_Paths"=w26:T19[])  [unwired: 10 in]
  n11 = call "Compute_Layer_Id_Patch_Permutationsvi.vi"("Max_#Layers_in_a_Group"="Max_Layers_In_Group", "Min_#Layers_in_a_Group"="Min_Layers_In_Group", "Patch_Sizes"="Patch Sizes", "Layer_IDs"="Layer ID") -> ("LayerID,PatchSize Permutations"=w23:T13[])  [unwired: 7 in]
  "Generated_Feature_Layers" <- w23
  n12 = Reverse 1D Array(array=w29) -> (reversed array=w28:sgl[])
  n13 = local write "dT_DS_Read(Train)"(w10) -> ()
  n14 = local write "dT_DS_Read(Test)"(w10) -> ()
  n15 = local write "dT_Init"(w10) -> ()
  n16 = local write "dT_Embed"(w10) -> ()
  n17 = local write "dT_Coreset"(w10) -> ()
  n18 = local write "dT_Predict"(w10) -> ()
  n19 = local write "dT_Eval"(w10) -> ()
  n20 = local write "Elapsed Time"(w10) -> ()
  n21 = Array To Spreadsheet String(delimiter (Tab)=",", array=w5, 3:"" ("spreadsheet string")) -> (spreadsheet string=w7:string)
  n22 = call <vilib>:"NN_Get_T_dT.vi"("error in"=w11) -> ("T_out"=w19:dbl, "error out"=w18:errorcluster)  [unwired: 6 in, 1 out]
  n23 = for {
    N -> [w69]
    tunnel: "Img Res. W" -> [w89]
    tunnel: "Proj._Dim." -> [w88]
    tunnel: w28 -> [w86]
    tunnel: w26 -> [w85]
    tunnel: w23 -> [w84]
    tunnel: w13 -> [w50] mode=indexing
    tunnel: "Destination_Path" -> [w60]
    tunnel: w12 -> [w71]
    shift-right: [w67] -> _
    shift-left: w20 -> [w68]
    tunnel: w19 -> [w66]
    tunnel: "Img Res. H" -> [w64]
    tunnel: w18 -> [w72]
    tunnel: [w43] -> w3
    tunnel: w7 -> [w46]
    i -> [w65]
    stop <- w63 stop-if-true
    w82 = ""  # Best_Params
    w83 = sgl 0.0  # Best_AUC
    w87 = 0  # Iteration
    n24 = local read "Single DS?"() -> (w61:bool)
    n25 = Build Path(base path=w60, name or relative path=w50) -> (appended path=w59:path)
    n26 = Build Path(base path=w71, name or relative path=w50) -> (appended path=w70:path)
    n27 = Concatenate Strings("Results_" ("string"), w50, ".csv" ("string")) -> (w52:string)
    n28 = Select(t=w60, s=w61, f=w59) -> (s? t:f=w49:path)
    n29 = Build Path(base path=w49, name or relative path=w52) -> (appended path=w56:path)
    n30 = Build Path(base path=w70, name or relative path="Train" ("String")) -> (appended path=w78:path)
    n31 = Build Path(base path=w70, name or relative path="Test" ("String")) -> (appended path=w76:path)
    n32 = Build Path(base path=w70, name or relative path="ground_truth" ("String")) -> (appended path=w77:path)
    n33 = Build Path(base path=w49, name or relative path="Images" ("String")) -> (appended path=w75:path)
    n34 = call <vilib>:"Create Directory Recursive.vi"("error in (no error)"=w72, "directory"=w75) -> ("error out"=w58:errorcluster, "directory copy"=w73:path)  [unwired: 3 in, 1 out]
    n35 = Open/Create/Replace File(file path (use dialog)=w56, error in=w58, operation (0:open)=T20."replace or create") -> (refnum out=w55:refnum<file>, error out=w54:errorcluster)  [unwired: 3 in, 1 out]
    n36 = Write to Text File(file (use dialog)=w55, text=w46, error in=w54) -> (refnum out=w47:refnum<file>, error out=w48:errorcluster)  [unwired: 1 in, 1 out]
    n37 = for "NNFE" {
      N -> [w103]
      tunnel: w89 -> [w116]
      tunnel: w77 -> [w115]
      tunnel: w88 -> [w114]
      tunnel: w76 -> [w113]
      tunnel: w78 -> [w112]
      tunnel: w73 -> [w111]
      tunnel: w66 -> [w110]
      tunnel: w84 -> [w109]
      tunnel: w86 -> [w107]
      tunnel: w85 -> [w105] mode=indexing
      shift-right: [w104] -> _
      shift-left: w87 -> [w108]
      shift-right: [w101] -> _
      shift-left: w83 -> [w102]
      shift-right: [w99] -> _
      shift-left: w82 -> [w100]
      shift-right: [w97] -> w67
      shift-left: w68 -> [w98]
      tunnel: w64 -> [w95]
      tunnel: w48 -> [w106]
      tunnel: [w93] -> w44
      tunnel: [w92] -> w62
      tunnel: w47 -> [w91]
      tunnel: [w90] -> w45
      i -> [w96]
      stop <- w94 stop-if-true
      n38 = for "Image Resolution" {
        N -> [w144]
        tunnel: w115 -> [w162]
        tunnel: w112 -> [w163]
        tunnel: w116 -> [w122] mode=indexing
        tunnel: w114 -> [w166]
        tunnel: w107 -> [w165]
        tunnel: w113 -> [w161]
        tunnel: w111 -> [w153]
        tunnel: w110 -> [w152]
        tunnel: w109 -> [w145]
        shift-right: [w142] -> w104
        shift-left: w108 -> [w143]
        tunnel: w105 -> [w136]
        shift-right: [w134] -> w101
        shift-left: w102 -> [w135]
        shift-right: [w132] -> w99
        shift-left: w100 -> [w133]
        shift-right: [w130] -> w97
        shift-left: w98 -> [w131]
        tunnel: w95 -> [w123] mode=indexing
        tunnel: w106 -> [w164]
        tunnel: [w121] -> w93
        tunnel: [w120] -> w92
        tunnel: w91 -> [w119]
        tunnel: [w118] -> w90
        i -> [w128]
        stop <- w141 stop-if-true
        w150 = u32 1 items=["Zero Order", "Bi-Linear", "Quadratic", "Cubic Spline"] ("Interpolation Type")
        w137 = string[] ["good", "Good", "normal", "OK"] ("Good Folder Name")
        n39 = Bundle By Name(cluster=T5 {"C"=3, "H"=0, "W"=0} ("Input_Dims"), "H"=w123, "W"=w122) -> (w146:T5)
        n40 = Bundle By Name(cluster=T21 {"DS_Name"="", "Input_Dims"={"C"=3, "H"=224, "W"=224}, "Cropping"={"Left"=-1.0, "Top"=-1.0, "Right"=-1.0, "Bottom"=-1.0}, "Interpolation Type"=1, "MultiStage_ReSample?"=FALSE, "Dataset_Stats"={"means"={"R"=0.5385, "G"=0.5348, "B"=0.551}, "stds"={"R"=0.3673, "G"=0.3673, "B"=0.3505}}} ("PreProcessing_Options"), "Input_Dims"=w146, "Interpolation Type"=w150, "MultiStage_ReSample?"=TRUE) -> (w139:T21)
        n41 = call "PatchCore_DS_Reader.vi"("Read Options"=T25 {"Read Bads?"=FALSE, "Read GTs?"=FALSE, "Update. DS Stats?"=TRUE}, "Good Unique Labels"=w137, "PreProc_Options_in"=w139, "error in"=w164, "Folder Path"=w163) -> ("error out"=w160:errorcluster, "PreProc_Options_out"=w138:T21, "Dataset"=w155:T27, "dT_DS_Reader"=w127:dbl)  [unwired: 3 in]
        "dT_DS_Read(Train)" <- w127
        n42 = call "Accumulator.vi"("in"=w127) -> ("accumulate_out"=→"dT_DS_Read(Train)":dbl)  [unwired: 10 in]
        n43 = call "PatchCore_DS_Reader.vi"("Read Options"=T25 {"Read Bads?"=TRUE, "Read GTs?"=TRUE, "Update. DS Stats?"=FALSE}, "Good Unique Labels"=w137, "PreProc_Options_in"=w138, "error in"=w160, "GT Folder Path"=w162, "Folder Path"=w161) -> ("error out"=w129:errorcluster, "Dataset"=w156:T27, "dT_DS_Reader"=w125:dbl)  [unwired: 2 in, 1 out]
        "dT_DS_Read(Test)" <- w125
        n44 = call "Accumulator.vi"("in"=w125) -> ("accumulate_out"=→"dT_DS_Read(Test)":dbl)  [unwired: 10 in]
        n45 = for "Feature_Layers" {
          N -> [w183]
          tunnel: w166 -> [w192]
          tunnel: w165 -> [w191]
          tunnel: w156 -> [w189]
          tunnel: w155 -> [w188]
          tunnel: w153 -> [w187]
          tunnel: w152 -> [w186]
          tunnel: w146 -> [w185]
          tunnel: w145 -> [w184] mode=indexing
          tunnel: [w182] -> w120
          shift-right: [w181] -> w142
          shift-left: w143 -> [w180]
          tunnel: w136 -> [w176]
          shift-right: [w174] -> w134
          shift-left: w135 -> [w175]
          shift-right: [w172] -> w132
          shift-left: w133 -> [w173]
          shift-right: [w170] -> w130
          shift-left: w131 -> [w171]
          tunnel: w129 -> [w190]
          tunnel: [w178] -> w140
          tunnel: w119 -> [w168]
          tunnel: [w167] -> w118
          i -> [w169]
          stop <- w179 stop-if-true
          n46 = Unbundle(w184) -> ("[LayerID, PatchSize]"=→"[LayerID, PatchSize]":cluster{"Layer_ID":i32, "Patch_Size":i32}[])
          n47 = for "Rand Proj Eps" {
            N -> [w235]
            tunnel: w188 -> [w246]
            tunnel: w192 -> [w241] mode=indexing
            tunnel: w191 -> [w196]
            tunnel: w189 -> [w244]
            tunnel: w187 -> [w243]
            tunnel: w186 -> [w242]
            tunnel: w185 -> [w237]
            tunnel: w184 -> [w236]
            tunnel: [w234] -> w182
            shift-right: [w232] -> w181
            shift-left: w180 -> [w233]
            tunnel: w176 -> [w219]
            shift-right: [w216] -> w174
            shift-left: w175 -> [w217]
            shift-right: [w214] -> w172
            shift-left: w173 -> [w215]
            shift-right: [w212] -> w170
            shift-left: w171 -> [w213]
            tunnel: w190 -> [w249]
            tunnel: [w230] -> w178
            tunnel: w168 -> [w203]
            tunnel: [w202] -> w167
            i -> [w210]
            stop <- w231 stop-if-true
            w225 = FALSE  # Destroy Embeds Afterwards?
            n48 = local read "DS Size(Train)"() -> (w193:i32)
            n49 = Bundle By Name(cluster="NNFE_CFG", "Feature_Layers"=w236) -> (w229:T11)
            n50 = Bundle By Name(cluster="NNPC_Setup", "Input_Dims"=w237) -> (w228:T4)
            n51 = Bundle By Name(cluster="Dim Reduction", "Target_Dim"=w241) -> (w201:T9)
            n52 = call <vilib>:"NNPC_Init(Train).vi"("error in"=w249, "NNFE_CFG"=w229, "NNPC_Setup"=w228, "NNFE_Paths"=w219) -> ("error out"=w247:errorcluster, "NNPC_out"=w194:T29, "dT_Init_Train"=w206:dbl)  [unwired: 5 in]
            "dT_Init" <- w206
            n53 = call "Convert_Coreset_Sizes_in_Percent_to_Number.vi"("input cluster"=w194, "DS_Size"=w193, "Coreset_Sizes in"=w196) -> ("Coreset_Sizes out"=w195:i32[])  [unwired: 8 in]
            n54 = Array Max & Min(array=w195) -> (max value=w221:i32)  [unwired: 3 out]
            n55 = Bundle By Name(cluster="Coreset_Params", "CoreSet_Size"=w221) -> (w200:T2)
            n56 = call "Accumulator.vi"("in"=w206) -> ("accumulate_out"=→"dT_Init":dbl)  [unwired: 10 in]
            n57 = call "Check_and_Update_Coreset_Params.vi"("NNPC_out"=w194, "DS_Size"=w193, "Coreset_Params in"=w200) -> ("Online_Coreset_Params out"=w198:T2, "Coreset_Params out"=w199:T2)  [unwired: 7 in]
            n58 = call-poly <vilib>:"NNPC_Generate_Embedding.vi"("Dataset"=w246, "Dim_Reduction"=w201, "error in"=w247, "Online_Coreset_Params"=w198, "NNPC_in"=w194) -> ("error out"=w224:errorcluster, "Feature_Embeddings"=w223:variant, "NNPC_out"=w222:T29, "dT_Embed"=w205:dbl)  [unwired: 2 in, 1 out]
            "dT_Embed" <- w205
            n59 = Unbundle By Name(w198) -> ("CoreSet_Size"=→"Online_CoreSet_Size":sgl)
            n60 = Unbundle By Name(w194) -> ("NN.Name"=→"Feature Extractor":string)
            n61 = call "Accumulator.vi"("in"=w205) -> ("accumulate_out"=→"dT_Embed":dbl)  [unwired: 10 in]
            n62 = call <vilib>:"NNPC_Generate_MemBank.vi"("Destroy Embeds Afterwards?"=w225, "Coreset_Params"=w199, "error in"=w224, "Feature_Embeddings"=w223, "NNPC_in"=w222) -> ("error out"=w211:errorcluster, "Max_Distances"=→"Max_Dist":sgl[], "NNPC_out"=w220:T29, "dT_Coreset"=w204:dbl)  [unwired: 2 in, 1 out]
            "dT_Coreset" <- w204
            n63 = call "Accumulator.vi"("in"=w204) -> ("accumulate_out"=→"dT_Coreset":dbl)  [unwired: 10 in]
            n64 = for "Coreset Size" {
              N -> [w302]
              shift-right: [w265] -> w248
              shift-left: w220 -> [w300]
              shift-right: [w296] -> w245
              shift-left: w211 -> [w299]
              tunnel: w244 -> [w310]
              tunnel: w243 -> [w305]
              tunnel: w242 -> [w304]
              tunnel: [w301] -> w234
              shift-right: [w291] -> w232
              shift-left: w233 -> [w266]
              tunnel: w195 -> [w298] mode=indexing
              shift-right: [w287] -> w216
              shift-left: w217 -> [w294]
              shift-right: [w288] -> w214
              shift-left: w215 -> [w293]
              shift-right: [w290] -> w212
              shift-left: w213 -> [w289]
              tunnel: w203 -> [w270]
              tunnel: [w267] -> w202
              i -> [w286]
              stop <- w301 stop-if-true
              w306 = TRUE  # Gen. FP Snapshot?
              n65 = call <vilib>:"NNPC_Shrink_MemBank.vi"("Coreset_Size"=w298, "error in"=w299, "NNPC_in"=w300) -> ("error out"=w276:errorcluster, "NNPC_out"=w277:T29)  [unwired: 7 in]
              n66 = local read "DS Size(Test)"() -> (w308:i32)
              n67 = call-poly <vilib>:"NNPC_Predict.vi"("Dataset"=w310, "Feature_Scorer_Params"="Feature_Scorer_Params", "error in"=w276, "NNPC_in"=w277) -> ("error out"=w313:errorcluster, "Anomaly_Maps"=w312:sgl[][][], "Pred_Scores"=w314:sgl[], "NNPC_out"=w315:T29, "dT_Predict"=w284:dbl)  [unwired: 3 in]
              "dT_Predict" <- w284
              n68 = Divide(x=w284, y=w308) -> (x/y=→"dT_Inference":dbl)
              n69 = call "Accumulator.vi"("in"=w284) -> ("accumulate_out"=→"dT_Predict":dbl)  [unwired: 10 in]
              n70 = call <vilib>:"NNPC_Eval.vi"("Eval_Config"=T26 {"Extract_Good_Pixels_from_Bad"=FALSE, "# bins"=100} ("Eval Config"), "Dataset"=w310, "error in"=w313, "Anomaly_Maps"=w312, "Pred_Scores"=w314, "NNPC_in"=w315) -> ("error out"=w275:errorcluster, "Evaluation_Metrics"=w250:T45, "NNPC_out"=w265:T29, "dT_Eval"=w282:dbl)  [unwired: 2 in]
              "dT_Eval" <- w282
              n71 = call "Accumulator.vi"("in"=w282) -> ("accumulate_out"=→"dT_Eval":dbl)  [unwired: 10 in]
              n72 = Unbundle By Name(w250) -> ("Evaluation_Metrics(Pixel)"=w255:T15, "Evaluation_Metrics(Image)"=w254:T15)
              n73 = flat-sequence {
                tunnel: w255 -> [w343]
                tunnel: w254 -> [w342]
                tunnel: [w353] -> w307
                tunnel: [w352] -> w303
                tunnel: [w351] -> w258
                tunnel: w265 -> [w350]
                tunnel: [w349] -> w264
                tunnel: [w348] -> w263
                tunnel: [w347] -> w262
                tunnel: [w346] -> w261
                tunnel: [w345] -> w260
                tunnel: [w344] -> w259
                frame #0 {
                  "Evaluation_Metrics(Image)" <- w342
                  "Evaluation_Metrics(Pixel)" <- w343
                }
                frame #1 {
                  n74 = local read "DS_Name"() -> (w347:string)
                  n75 = local read "Feature Extractor"() -> (w351:string)
                  n76 = local read "DS Size(Train)"() -> (w346:i32)
                  n77 = local read "Coreset Size"() -> (w345:i32)
                  n78 = local read "Proj. Dim."() -> (w344:i32)
                  n79 = local read "dT_Inference"() -> (w352:dbl)
                  n80 = local read "dT_Init"() -> (w356:dbl)
                  n81 = local read "dT_Embed"() -> (w355:dbl)
                  n82 = local read "dT_Coreset"() -> (w354:dbl)
                  n83 = Unbundle By Name(w350) -> ("NN.Dims_In.H"=w349:i32, "NN.Dims_In.W"=w348:i32)
                  n84 = Compound Arithmetic op=ADD(w356, w355, w354) -> (w353:dbl)
                }
              }
              n85 = flat-sequence {
                frame #0 {
                  n86 = local read "Img Res. H"() -> (w329:i32[])
                  n87 = local read "Generated_Feature_Layers"() -> (w335:T13[])
                  n88 = local read "Proj._Dim."() -> (w341:i32[])
                  n89 = local read "Coreset_Size"() -> (w340:sgl[])
                  n90 = local read "NNFE_Folder_Paths"() -> (w334:path[])
                  n91 = local read "DS"() -> (w330:i32)
                  n92 = Array Size(array=w329) -> (size(s)=w338:i32)
                  n93 = Array Size(array=w335) -> (size(s)=w339:i32)
                  n94 = Array Size(array=w341) -> (size(s)=w337:i32)
                  n95 = Array Size(array=w340) -> (size(s)=w336:i32)
                  n96 = Array Size(array=w334) -> (size(s)=w333:i32)
                  n97 = Compound Arithmetic op=MULTIPLY(w338, w339, w337, w336, w333) -> (w332:i32)
                  "Tot Itr of one DS" <- w332
                  n98 = Multiply(x=w332, y=w330) -> (x*y=→"Total Iters":i32)
                }
              }
              n99 = local read "[LayerID, PatchSize]"() -> (w251:T18)
              n100 = Bundle By Name(cluster=T1 {"Idx"=0, "Name"="", "Feature Extractor"="wrn_50_2_2_bnmerge", "Layers"="", "DS_Size"=0, "H"=0, "W"=-1, "Coreset Size"=0, "Proj_Dim"=0, "Good_Max(Img)"=0.0, "Bad_Min(Img)"=0.0, "Rel_Margin"=0.0, "Image_AUC"=0.0, "Pixel_AUC"=0.0, "Image_F1_Max"=0.0, "Pixel_F1_Max"=0.0, "Train_Time"=0.0, "Inf_Time"=0.0} ("Model_Info_and_Report"), "Idx"=w266, "Name"=w262, "Feature Extractor"=w258, "DS_Size"=w261, "Coreset Size"=w260, "Proj_Dim"=w259, "Inf_Time"=w303, "Train_Time"=w307, "H"=w264, "W"=w263) -> (w253:T1)
              n101 = flat-sequence {
                tunnel: w252 -> [_]
                tunnel: [w317] -> w279
                frame #0 {
                  n102 = local read "Evaluation_Metrics(Image)"() -> (w317:T15)
                }
              }
              n103 = Equal To 0?(x=w266) -> (x = 0?=w281:bool)
              n104 = call "Model_Info_and_Report_Write_Eval_Layer_Info.vi"("Evaluation_Metrics"=w250, "[LayerID, PatchSize]"=w251, "Model_Info_and_Report in"=w253) -> ("Model_Info_and_Report out"=w252:T1)  [unwired: 8 in]
              n105 = call <vilib>:"NN_Get_T_dT.vi"("T_in"=w304, "error in"=w275) -> ("error out"=w269:errorcluster, "dT"=→"Elapsed Time" →"Elapsed Time":dbl)  [unwired: 5 in, 1 out]
              n106 = call "Generate_Model_Info(CSV).vi"("Model_Info_and_Report"=w252) -> ("Model_Info(CSV)"=w256:string)  [unwired: 10 in]
              n107 = Unbundle By Name(w279) -> ("Eval Stats.AUROC"=w278:sgl)
              n108 = call "Geneate_Model_Name.vi"("Model_Info_and_Report"=w252) -> ("Model_Name"=w257:string)  [unwired: 10 in]
              n109 = case shown="False" w281 {
                tunnel: [w324 w326] -> w295
                tunnel: w278 -> [w323 w326]
                tunnel: w294 -> [w322 _]
                tunnel: w257 -> [w320 w325]
                tunnel: w293 -> [w319 _]
                tunnel: [w318 w325] -> w292
                frame False {
                  n110 = Greater?(x=w323, y=w322) -> (0:w321:bool)
                  n111 = Select(t=w323, s=w321, f=w322) -> (s? t:f=w324:sgl)
                  n112 = Select(t=w320, s=w321, f=w319) -> (s? t:f=w318:string)
                }
                frame True {
                }
              }
              n113 = Set File Position(refnum=w270, from (0:start)=enum16{"start", "end", "current"}."end", error in=w269) -> (refnum out=w273:refnum<file>, error out=w272:errorcluster)  [unwired: 1 in]
              n114 = Write to Text File(file (use dialog)=w273, text=w256, error in=w272) -> (refnum out=w267:refnum<file>, error out=w268:errorcluster)  [unwired: 1 in, 1 out]
              n115 = case shown="True" w306 {
                tunnel: w305 -> [_ w361]
                tunnel: w268 -> [w357 w364]
                tunnel: [w357 w363] -> w296
                tunnel: w257 -> [_ w359]
                frame False {
                }
                frame True {
                  n116 = Concatenate Strings(w359, ".png" ("string")) -> (w358:string)
                  n117 = control-ref of="Tab Control"() -> (w365:refnum<vi>)
                  n118 = Build Path(base path=w361, name or relative path=w358) -> (appended path=w362:path)
                  n119 = call "Generate_FP_Snapshot.vi"("TabControl in"=w365, "error in"=w364, "File_Name"=w362) -> ("error out"=w363:errorcluster)  [unwired: 8 in]
                }
              }
              n120 = flat-sequence {
                tunnel: w295 -> [w328]
                tunnel: w292 -> [w327]
                tunnel: [w328] -> w287
                tunnel: [w327] -> w288
                frame #0 {
                  "Best_Model" <- w327
                  "Best_AUC" <- w328
                }
              }
              n121 = Increment(x=w289) -> (x+1=w290:i32)
              n122 = Increment(x=w266) -> (x+1=w291:i32)
              n123 = Or(x=w296, y="Stop") -> (x .or. y?=w301:bool)
              "Coreset Size" <- w286
              "Coreset Size" <- w302
              "Current Iter" <- w289
              "Coreset Size" <- w298
              "Crrnt Iter" <- w266
            }
            n124 = call <vilib>:"NNPC_Destroy.vi"("error in"=w245, "NNPC_in"=w248) -> ("error out"=w230:errorcluster)  [unwired: 9 in]
            n125 = Or(x=w230, y=w234) -> (x .or. y?=w231:bool)
            "Proj. Dim." <- w210
            "Proj. Dim." <- w241
            "Proj. Dim." <- w235
          }
          n126 = Or(x=w178, y=w182) -> (x .or. y?=w179:bool)
          "Feature_Layers" <- w169
          "Feature_Layers" <- w183
        }
        n127 = Unbundle By Name(w156) -> ("Dataset_Size"=→"DS Size(Test)":i32)
        n128 = Unbundle By Name(w155) -> ("Dataset_Size"=→"DS Size(Train)":i32)
        n129 = call-poly <vilib>:"NN_Dataset_Destroy.vi"("error in (no error)"=w140, "Dataset(In3D_Out3D)"=w156) -> ("error out"=w159:errorcluster)  [unwired: 9 in]
        n130 = call-poly <vilib>:"NN_Dataset_Destroy.vi"("error in (no error)"=w140, "Dataset(In3D_Out3D)"=w155) -> ("error out"=w154:errorcluster)  [unwired: 9 in]
        n131 = Merge Errors(w159, w154) -> (w121:errorcluster)
        n132 = Or(x=w120, y=w121) -> (x .or. y?=w141:bool)
        "Img Res." <- w128
        "Img._H" <- w123
        "Img Res." <- w144
        "Img._W" <- w122
      }
      n133 = Or(x=w92, y=w93) -> (x .or. y?=w94:bool)
      "NNFE" <- w103
      "NNFE" <- w96
    }
    n134 = Close File(refnum=w45, error in=w44) -> (error out=w43:errorcluster)  [unwired: 1 out]
    n135 = Or(x=w62, y=w43) -> (x .or. y?=w63:bool)
    "DS" <- w69
    "DS" <- w65
    "DS_Name" <- w50
  }
  n136 = local read "Single DS?"() -> (w1:bool)
  n137 = case shown="False" w1 {
    tunnel: "Destination_Path" -> [w368 _]
    tunnel: w3 -> [w367 w369]
    tunnel: [w366 w369] -> w2
    frame False {
      n138 = call "Generate_Best_of_Each_DS_Report.vi"("error in (no error)"=w367, "Destination_Path"=w368) -> ("error out"=w366:errorcluster)  [unwired: 9 in]
    }
    frame True {
    }
  }
  "error out" <- w2
